vi "Shutdown.vi"(8 "error in":errorcluster, 11 "Network Master in":refnum<class "Network Master.lvclass">) -> (0 "error out":errorcluster)   [LabVIEW 2021, in "Network Master.lvclass"]
doc: "This provides an interface for the master to close a connection to the slave."
uses:
  Network Master.lvclass
  Network Master.lvclass/Network Master.ctl
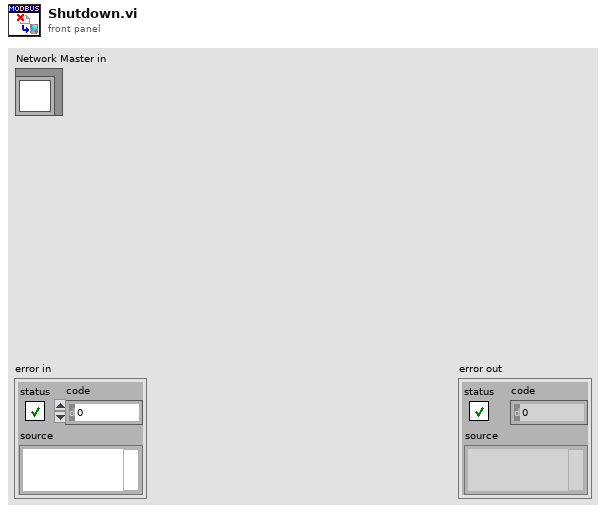
[diagram p1: front panel]
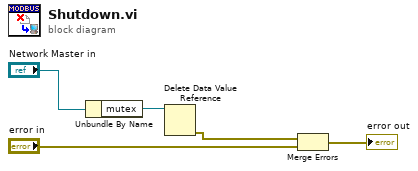
[diagram p0: block diagram]
diagram:
  n1 = Unbundle By Name("Network Master in") -> ("mutex"=w4:refnum<data-value>)
  n2 = Delete Data Value Reference(data value reference=w4) -> (error out=w2:errorcluster)  [unwired: 1 in, 1 out]
  n3 = Merge Errors(w2, "error in") -> (→"error out":errorcluster)
